vi "HolDrvCtrl_PackProfPID.vi"(6 "Period":dbl=0.02, 8 "Max Accel":dbl format="%20.4f", 9 "Max Speed":dbl format="%20.4f", 10 "PID Input Limits":T1={"MaxInput"=3.141592653589793, "MinInput"=-3.141592653589793, "Continuous"=TRUE} {"MinInput" format="%#_13g"; "MaxInput" format="%#_13g"}, 11 "Theta PID Tuning":T6={"Kp"=0.0, "Ki"=0.0, "Kd"=0.0, "MaximumIntegral"=9.9e+30, "MinimumIntegral"=-9.9e+30}) -> (3 "Theta PID CONTROLLER":T2={"Controller"={"Kp"=0.0, "Ki"=0.0, "Kd"=0.0, "Period"=0.0, "Max_Integral"=1.0, "Min_Integral"=-1.0, "Max_Input"=0.0, "Min_Input"=0.0, "Continuous"=FALSE, "PositionError"=0.0, "VelocityError"=0.0, "PrevError"=0.0, "TotalError"=0.0, "PositionTolerance"=0.05, "VelocityTolerance"=9.99e+35, "SetPoint"=0.0, "Kf"=0.0, "Prev_Deriv"=0.0, "Prev_Deriv 2"=0.0, "DerivativeFilter"=FALSE, "Min_Output"=-9.99e+35, "Max_Output"=9.9e+35, "Prev_F_P"=0.0, "Prev_F_P_2"=0.0, "AntiWindupActive"=FALSE, "Measurement"=0.0}, "Goal"={"Position"=0.0, "Velocity"=0.0}, "Setpoint"={"Position"=0.0, "Velocity"=0.0}, "Constraint"={"MaxVelocity"=0.0, "MaxAcceleration"=0.0}} {"Constraint"."MaxAcceleration" format="%16_6e"; "Constraint"."MaxVelocity" format="%16_6e"; "Setpoint"."Velocity" format="%16_6e"; "Setpoint"."Position" format="%16_6e"; "Goal"."Velocity" format="%16_6e"; "Goal"."Position" format="%16_6e"; "Controller"."Measurement" format="%16_6e"; "Controller"."Prev_F_P_2" format="%16_6e"; "Controller"."Prev_F_P" format="%16_6e"; "Controller"."Max_Output" format="%16_6e"; "Controller"."Min_Output" format="%16_6e"; "Controller"."Prev_Deriv 2" format="%16_6e"; "Controller"."Prev_Deriv" format="%16_6e"; "Controller"."Kf" format="%16_6e"; "Controller"."SetPoint" format="%16_6e"; "Controller"."VelocityTolerance" format="%16_6e"; "Controller"."PositionTolerance" format="%16_6e"; "Controller"."TotalError" format="%16_6e"; "Controller"."PrevError" format="%16_6e"; "Controller"."VelocityError" format="%16_6e"; "Controller"."PositionError" format="%16_6e"; "Controller"."Min_Input" format="%16_6e"; "Controller"."Max_Input" format="%16_6e"; "Controller"."Min_Integral" format="%16_6e"; "Controller"."Max_Integral" format="%16_6e"; "Controller"."Period" format="%16_6e"; "Controller"."Kd" format="%16_6e"; "Controller"."Ki" format="%16_6e"; "Controller"."Kp" format="%16_6e"})   [LabVIEW 2019, in "Trajectory_Library.lvlib"]
doc: "Convience, single call, LabVIEW function. Packs the tuning parameters of the Theta Profiled PID controller used by the Holonomic Controller. \n\nNOTE -- This version does NOT support dynamic tuning. The constants are read only used during the first execution cycle.\n \nInputs:\n - PID Tuning -- PID Tuning parameters containing:\n - Kp -- The proportional coefficient.\n - Ki -- The integral coefficient.\n - Kd -- The derivative coefficient.\n - Maximum Integral -- The maximum value of the integrator.\n - Minimum Integral -- The minimum value of the integrator.\n - PID Input Limits -- Cluster containing:\n - MaxInput -- (Default: 0)\n - MinInput -- (Default: 0)\n - Continous -- When True indicates that the input is continuous. (Default: False)\n - Max_Speed -- Maximum speed robot rotation\n - Max_Accel -- Maximum acceleration of robot rotation.\n - Period -- Period of repeated calls in seconds. (Default: 0.020)\n\nOutputs:\n - Theta Profiled_PID_Controller -- Created Theta Profiled PID_Controller data cluster"
uses:
  Trajectory_Library.lvlib
  TypeDef/PID_CONTROLLER.ctl
  TypeDef/PID_TUNING.ctl
  TypeDef/TRAPEZOID_PROFILE_STATE.ctl
  TypeDef/TRAPEZOID_PROFILE_CONSTRAINT.ctl
  TypeDef/PROFILED_PID_CONTROLLER.ctl
  TypeDef/PID_INPUT_LIMITS.ctl
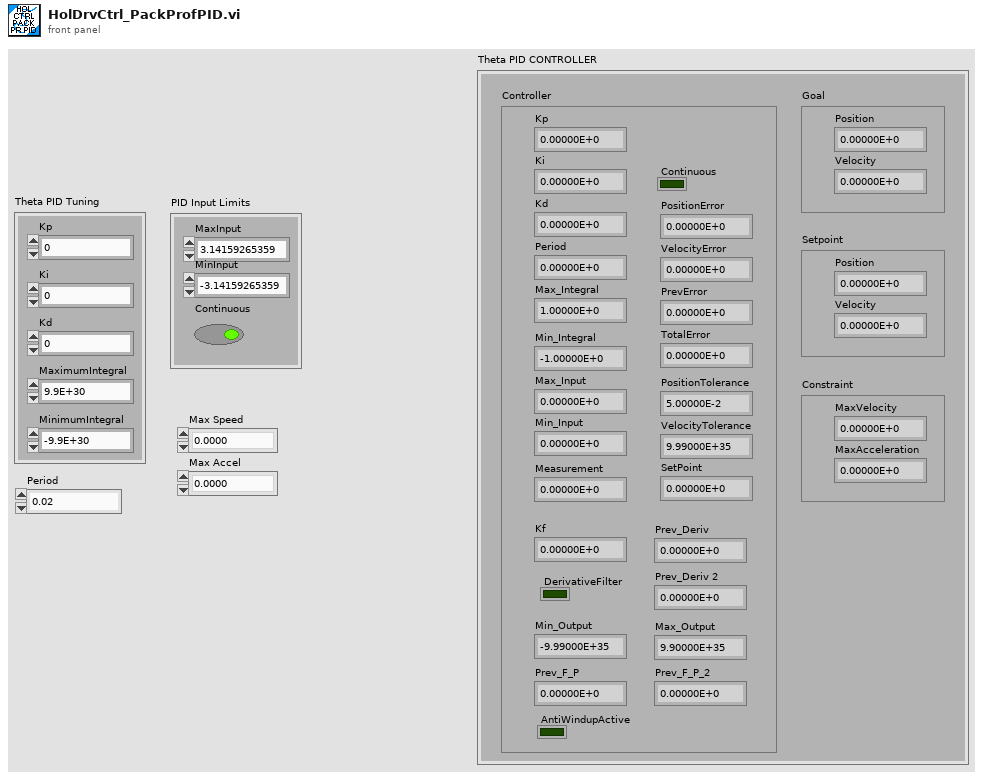
[diagram p1: front panel]
types:
  T1 = typedef "Trajectory_Library.lvlib/PID_INPUT_LIMITS.ctl" = cluster{"MaxInput":dbl, "MinInput":dbl, "Continuous":bool}
  T2 = typedef "Trajectory_Library.lvlib/PROFILED_PID_CONTROLLER.ctl" = cluster{"Controller":T3, "Goal":T4, "Setpoint":T4, "Constraint":T5}
  T3 = typedef "Trajectory_Library.lvlib/PID_CONTROLLER.ctl" = cluster{"Kp":dbl, "Ki":dbl, "Kd":dbl, "Period":dbl, "Max_Integral":dbl, "Min_Integral":dbl, "Max_Input":dbl, "Min_Input":dbl, "Continuous":bool, "PositionError":dbl, "VelocityError":dbl, "PrevError":dbl, "TotalError":dbl, "PositionTolerance":dbl, "VelocityTolerance":dbl, "SetPoint":dbl, "Kf":dbl, "Prev_Deriv":dbl, "Prev_Deriv 2":dbl, "DerivativeFilter":bool, "Min_Output":dbl, "Max_Output":dbl, "Prev_F_P":dbl, "Prev_F_P_2":dbl, "AntiWindupActive":bool, "Measurement":dbl}
  T4 = typedef "Trajectory_Library.lvlib/TRAPEZOID_PROFILE_STATE.ctl" = cluster{"Position":dbl, "Velocity":dbl}
  T5 = typedef "Trajectory_Library.lvlib/TRAPEZOID_PROFILE_CONSTRAINT.ctl" = cluster{"MaxVelocity":dbl, "MaxAcceleration":dbl}
  T6 = typedef "Trajectory_Library.lvlib/PID_TUNING.ctl" = cluster{"Kp":dbl, "Ki":dbl, "Kd":dbl, "MaximumIntegral":dbl, "MinimumIntegral":dbl}
  T7 = typedef "WPILib_Math.lvlib/TRAPEZOID_PROFILE_CONSTRAINT.ctl" = cluster{"MaxVelocity":dbl, "MaxAcceleration":dbl}
  T8 = typedef "WPILib_Math.lvlib/PROFILED_PID_CONTROLLER.ctl" = cluster{"Controller":T9, "Goal":T10, "Setpoint":T10, "Constraint":T7}
  T9 = typedef "WPILib_Math.lvlib/PID_CONTROLLER.ctl" = cluster{"Kp":dbl, "Ki":dbl, "Kd":dbl, "Period":dbl, "Max_Integral":dbl, "Min_Integral":dbl, "Max_Input":dbl, "Min_Input":dbl, "Continuous":bool, "PositionError":dbl, "VelocityError":dbl, "PrevError":dbl, "TotalError":dbl, "PositionTolerance":dbl, "VelocityTolerance":dbl, "SetPoint":dbl, "Kf":dbl, "Prev_Deriv":dbl, "Prev_Deriv 2":dbl, "DerivativeFilter":bool, "Min_Output":dbl, "Max_Output":dbl, "Prev_F_P":dbl, "Prev_F_P_2":dbl, "AntiWindupActive":bool, "Measurement":dbl}
  T10 = typedef "WPILib_Math.lvlib/TRAPEZOID_PROFILE_STATE.ctl" = cluster{"Position":dbl, "Velocity":dbl}
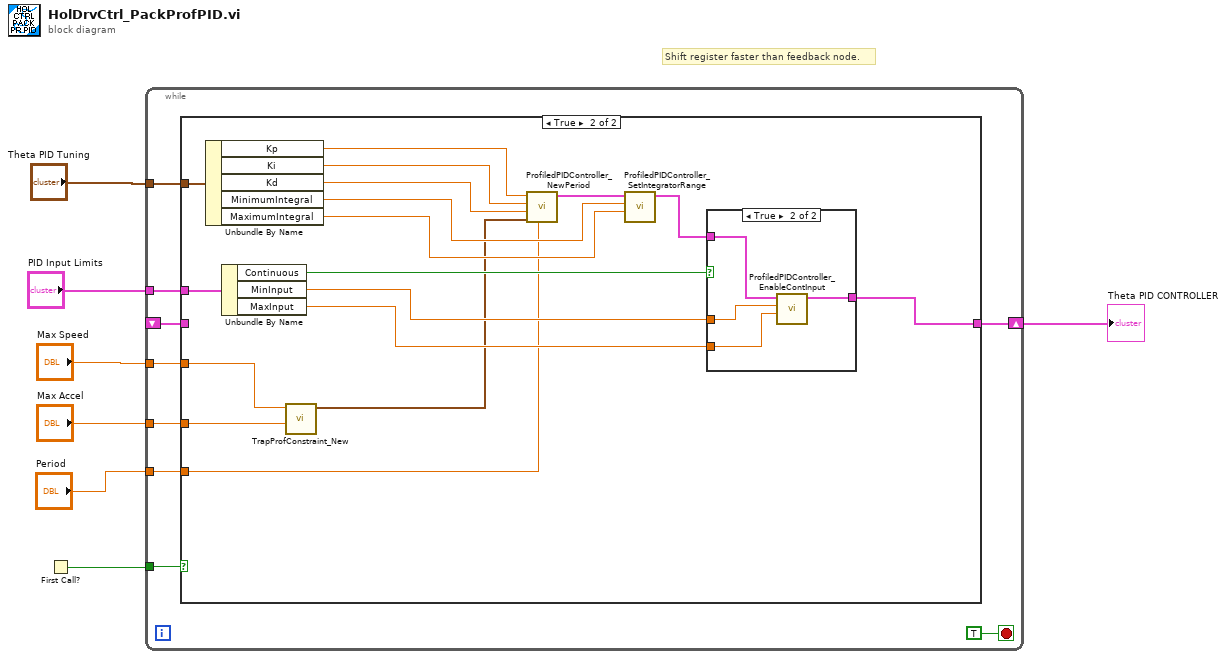
[diagram p0: block diagram]
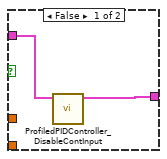
[diagram p3: hidden frame]
diagram:
  # "Shift register faster than feedback node."
  n1 = First Call?() -> (First Call?: T/F=w5:bool)
  n2 = while {
    tunnel: "Theta PID Tuning" -> [w16]
    tunnel: "Period" -> [w15]
    tunnel: w5 -> [w14]
    tunnel: "PID Input Limits" -> [w12]
    tunnel: "Max Speed" -> [w11]
    tunnel: "Max Accel" -> [w10]
    shift-right: [w13] -> w4
    shift-left: _ -> [w8]
    stop <- TRUE stop-if-true
    n3 = case shown="True" w14 {
      tunnel: w16 -> [_ w34]
      tunnel: [w17 w18] -> w13
      tunnel: w15 -> [_ w19]
      tunnel: w12 -> [_ w27]
      tunnel: w11 -> [_ w22]
      tunnel: w10 -> [_ w21]
      tunnel: w8 -> [w17 _]
      frame False {
      }
      frame True {
        n4 = Unbundle By Name(w34) -> ("Kp"=w33:dbl, "Ki"=w32:dbl, "Kd"=w31:dbl, "MinimumIntegral"=w29:dbl, "MaximumIntegral"=w28:dbl)
        n5 = Unbundle By Name(w27) -> ("Continuous"=w26:bool, "MinInput"=w24:dbl, "MaxInput"=w23:dbl)
        n6 = call "TrapProfConstraint_New.vi"("Max Accel"=w21, "Max Speed (M/S)"=w22) -> ("TRAPEZOID_PROFILE_CONSTRAINT"=w20:T7)  [unwired: 9 in]
        n7 = call "ProfiledPIDController_NewPeriod.vi"("Period"=w19, "Constraints"=w20, "Kd"=w31, "Ki"=w32, "Kp"=w33) -> ("PROFILED_PID_CONTROLLER"=w30:T2)  [unwired: 6 in]
        n8 = call "ProfiledPIDController_SetIntegratorRange.vi"("Maximum"=w28, "Minimum"=w29, "in PROFILED_PID_CONTROLLER"=w30) -> ("out PROFILED_PID_CONTROLLER"=w25:T8)  [unwired: 8 in]
        n9 = case shown="True" w26 {
          tunnel: w25 -> [w36 w40]
          tunnel: [w35 w39] -> w18
          tunnel: w24 -> [_ w38]
          tunnel: w23 -> [_ w37]
          frame False {
            n10 = call "ProfiledPIDController_DisableContInput.vi"("in PROFILED_PID_CONTROLLER"=w36) -> ("out PROFILED_PID_CONTROLLER"=w35:T2)  [unwired: 10 in]
          }
          frame True {
            n11 = call "ProfiledPIDController_EnableContInput.vi"("MaxInput"=w37, "MinInput"=w38, "in PROFILED_PID_CONTROLLER"=w40) -> ("out PROFILED_PID_CONTROLLER"=w39:T8)  [unwired: 8 in]
          }
        }
      }
    }
  }
  "Theta PID CONTROLLER" <- w4
